vi "Demo.vi"() -> ()   [LabVIEW 2017]
uses:
  <vilib>/picture/3D Picture Control/NI_3D Picture Control.lvlib
panel:
  out "3D Picture":refnum<vi>(3d-picture)
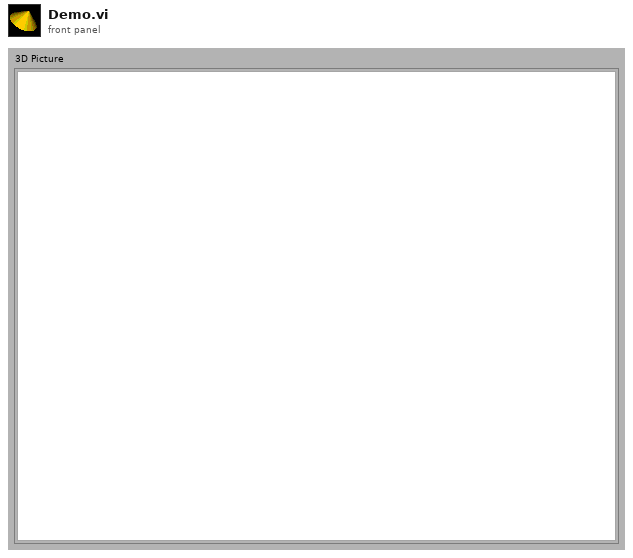
[diagram p1: front panel]
types:
  T1 = cluster{"Text":string, "Color Box":u32, "Alpha":sgl}
  T2 = cluster{"Height":sgl, "Radius":sgl, "Alpha":sgl, "Color Box":u32, "Detail":sgl}
  T3 = cluster{"Radius":sgl, "Color Box":u32, "Alpha":sgl, "Detail":sgl}
  T4 = cluster{"Height":sgl, "Radius":sgl, "Color Box":u32, "Alpha":sgl, "Detail":sgl}
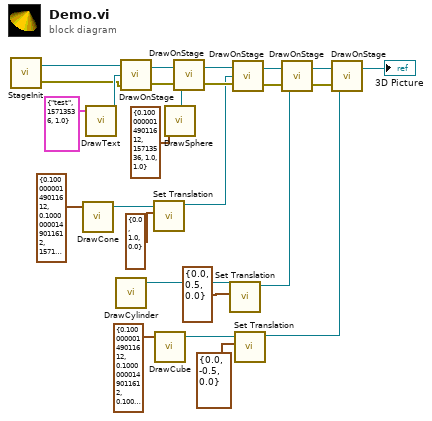
[diagram p0: block diagram]
diagram:
  n1 = call <userlib>:"StageInit.vi"() -> ("error out"=w18:errorcluster, "Stage out"=w19:refnum<vi>)  [unwired: 3 in]
  n2 = call <userlib>:"DrawCone.vi"("Cone"=T4 {"Height"=0.1, "Radius"=0.1, "Color Box"=15713536, "Alpha"=1.0, "Detail"=1.0}) -> ("object out"=w12:refnum<vi>)  [unwired: 5 in, 1 out]
  n3 = call <userlib>:"DrawText.vi"("Text"=T1 {"Text"="test", "Color Box"=15713536, "Alpha"=1.0}) -> ("object out"=w20:refnum<vi>)  [unwired: 5 in, 1 out]
  n4 = call <userlib>:"DrawCylinder.vi"() -> ("object out"=w24:refnum<vi>)  [unwired: 6 in, 1 out]
  n5 = call <userlib>:"DrawOnStage.vi"("error in"=w18, "object in"=w20, "Stage in"=w19) -> ("error out"=w17:errorcluster, "Stage out"=w16:refnum<vi>)
  n6 = call <vilib>:"Set Translation.vi"("Translation"=cluster{"X":sgl, "Y":sgl, "Z":sgl} {"X"=0.0, "Y"=1.0, "Z"=0.0}, "Scene Object"=w12) -> ("Translated Object"=w11:refnum<vi>)  [unwired: 8 in, 1 out]
  n7 = call <userlib>:"DrawCube.vi"("Cube"=T2 {"Height"=0.1, "Radius"=0.1, "Alpha"=0.1, "Color Box"=15713536, "Detail"=1.0} ("Cone")) -> ("object out"=w5:refnum<vi>)  [unwired: 5 in, 1 out]
  n8 = call <userlib>:"DrawSphere.vi"("Sphere"=T3 {"Radius"=0.1, "Color Box"=15713536, "Alpha"=1.0, "Detail"=1.0} ("Cone")) -> ("object out"=w1:refnum<vi>)  [unwired: 5 in, 1 out]
  n9 = call <userlib>:"DrawOnStage.vi"("error in"=w17, "object in"=w1, "Stage in"=w16) -> ("error out"=w15:errorcluster, "Stage out"=w14:refnum<vi>)
  n10 = call <vilib>:"Set Translation.vi"("Translation"=cluster{"X":sgl, "Y":sgl, "Z":sgl} {"X"=0.0, "Y"=0.5, "Z"=0.0}, "Scene Object"=w24) -> ("Translated Object"=w8:refnum<vi>)  [unwired: 8 in, 1 out]
  n11 = call <userlib>:"DrawOnStage.vi"("error in"=w15, "object in"=w11, "Stage in"=w14) -> ("error out"=w10:errorcluster, "Stage out"=w9:refnum<vi>)
  n12 = call <vilib>:"Set Translation.vi"("Translation"=cluster{"X":sgl, "Y":sgl, "Z":sgl} {"X"=0.0, "Y"=-0.5, "Z"=0.0}, "Scene Object"=w5) -> ("Translated Object"=w4:refnum<vi>)  [unwired: 8 in, 1 out]
  n13 = call <userlib>:"DrawOnStage.vi"("error in"=w10, "object in"=w8, "Stage in"=w9) -> ("error out"=w3:errorcluster, "Stage out"=w7:refnum<vi>)
  n14 = call <userlib>:"DrawOnStage.vi"("error in"=w3, "object in"=w4, "Stage in"=w7) -> ("Stage out"=→"3D Picture":refnum<vi>)  [unwired: 1 out]
